vi "Test DI and DO.vi"() -> ()   [LabVIEW 2013]
uses:
  SLL DAQ Engine/Software/Source Code/Sub VIs/DAQ Engine/Controls/SLL DE List of Digital Inputs.ctl
  SLL DAQ Engine/Software/Source Code/Sub VIs/DAQ Engine/Controls/SLL DE List of Digital Outputs.ctl
  Controls/ALTS-2015 LV2GBL Station Info Options.ctl
  SLL DAQ Engine/Software/Source Code/Sub VIs/DAQ Engine/Controls/SLL DE DI Global Options.ctl
  SLL DAQ Engine/Software/Source Code/Sub VIs/DAQ Engine/Controls/SLL DE DO Global Options.ctl
panel:
  out "Station Number":string
  in  "PC_ACK_Read_Tags":dbl
  out "Test Type":i32
  out "DO Channel Name":T1
  out "String":string
  in  "Invalid_SNo":dbl
  in  "Station_No_Start_Stop_Test":dbl
  in  "Start_Test":dbl
  in  "Rerun":dbl
  in  "Station_Number":dbl
  in  "Test_Result":dbl
  in  "Serial_Flange_Size":string
  in  "Serial_Displacement_Size":dbl
  in  "Serial_Adapter_Size":dbl
  in  "New_Serial":dbl
  in  "Scan_Trigger":dbl
  in  "Stop_Test":dbl
  in  "Task_Available_for_Robot":dbl
  in  "Robot_Available":dbl
  in  "DI Array":bool[](array[boolean])=[FALSE, FALSE, FALSE, FALSE, FALSE, FALSE, FALSE, FALSE, FALSE, FALSE, FALSE, FALSE, FALSE, FALSE, FALSE, FALSE, FALSE, FALSE, FALSE, FALSE, FALSE, FALSE, FALSE, FALSE, FALSE, FALSE, FALSE, FALSE]
  in  "DI Channel Name Array":T2[](array[typedef])=[enum."STATION1_START", enum."STATION1_STOP", enum."STATION1_CLAMPED", enum."STATION1_TC_PASS", enum."STATION1_TC_FAIL", enum."STATION1_TTA", enum."STATION1_TTB", enum."STATION2_START", enum."STATION2_STOP", enum."STATION2_CLAMPED", enum."STATION2_TC_PASS", enum."STATION2_TC_FAIL", enum."STATION2_TTA", enum."STATION2_TTB", enum."STATION3_START", enum."STATION3_STOP", enum."STATION3_CLAMPED", enum."STATION3_TC_PASS", enum."STATION3_TC_FAIL", enum."STATION3_TTA", enum."STATION3_TTB", enum."STATION4_START", enum."STATION4_STOP", enum."STATION4_CLAMPED", enum."STATION4_TC_PASS", enum."STATION4_TC_FAIL", enum."STATION4_TTA", enum."STATION4_TTB"]
  out "DO Channel Name Array":T1[](array[typedef])=[enum."STATION1_START TEST", enum."STATION1_STOP TEST", enum."STATION1_LIGHT1", enum."STATION1_LIGHT2", enum."STATION1_LIGHT3", enum."STATION1_SELECT_TEST", enum."STATION2_START TEST", enum."STATION2_STOP TEST", enum."STATION2_LIGHT1", enum."STATION2_LIGHT2", enum."STATION2_LIGHT3", enum."STATION2_SELECT_TEST", enum."STATION3_START TEST", enum."STATION3_STOP TEST", enum."STATION3_LIGHT1", enum."STATION3_LIGHT2", enum."STATION3_LIGHT3", enum."STATION3_SELECT_TEST", enum."STATION4_START TEST", enum."STATION4_STOP TEST", enum."STATION4_LIGHT1", enum."STATION4_LIGHT2", enum."STATION4_LIGHT3", enum."STATION4_SELECT_TEST"]
  out "DO Status":bool[](array[boolean])
  out "error out":errorcluster
  in  "error in":errorcluster
  in  "DI Channel Name":T2
  in  "stop":bool
  # "Simulation VI to send DI Status and reads the DO output"
  # "Write Tags\nPC Writes to PLC\nPLC can only read these tags"
  # "Read Tags\nPC Reads from PLC"
  # "Test Type1: TTA:1, TTB: 0;\nTest Type2: TTA:0, TTB: 1;\nTest Type3: TTA:1, TTB: 1;\nTest Type4: TTA:0, TTB: 0;"
  # "IDLE : \t\t100\nTest Running:\t 010\nPass\t\t110\nFail\t\t101"
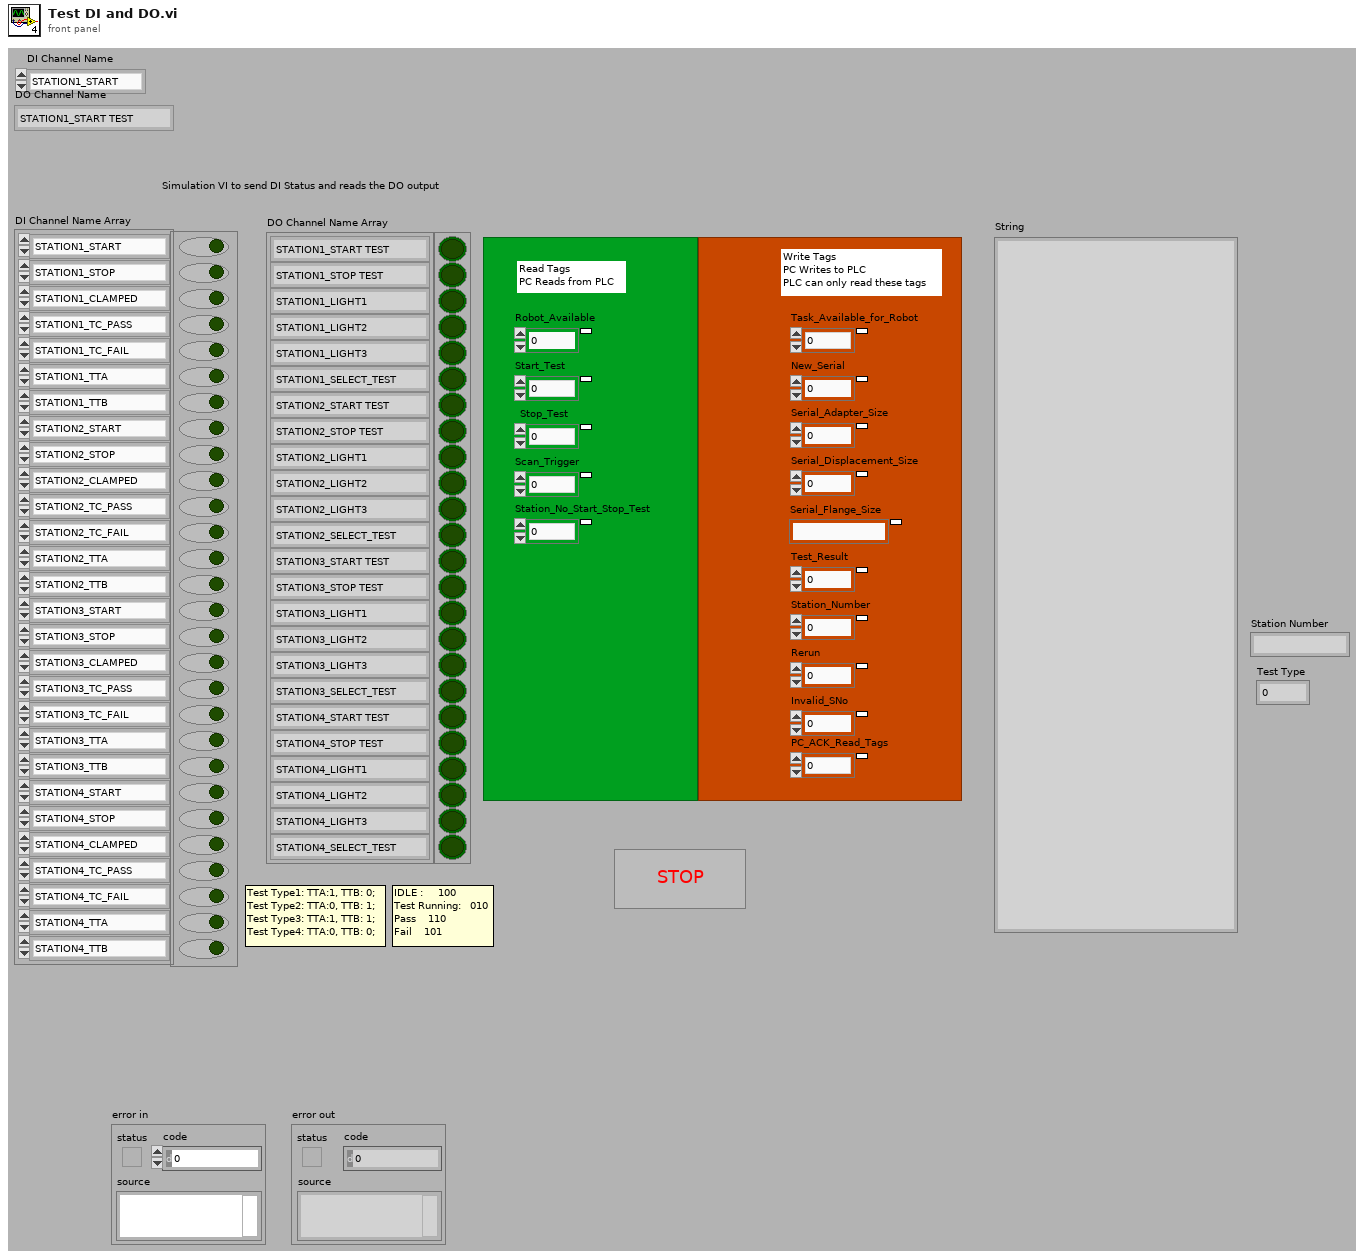
[diagram p1: front panel]
types:
  T1 = typedef "SLL DE List of Digital Outputs.ctl" = enum16{"STATION1_START TEST", "STATION1_STOP TEST", "STATION1_LIGHT1", "STATION1_LIGHT2", "STATION1_LIGHT3", "STATION1_SELECT_TEST", "STATION2_START TEST", "STATION2_STOP TEST", "STATION2_LIGHT1", "STATION2_LIGHT2", "STATION2_LIGHT3", "STATION2_SELECT_TEST", "STATION3_START TEST", "STATION3_STOP TEST", "STATION3_LIGHT1", "STATION3_LIGHT2", "STATION3_LIGHT3", "STATION3_SELECT_TEST", "STATION4_START TEST", "STATION4_STOP TEST", "STATION4_LIGHT1", "STATION4_LIGHT2", "STATION4_LIGHT3", "STATION4_SELECT_TEST"}
  T2 = typedef "SLL DE List of Digital Inputs.ctl" = enum16{"STATION1_START", "STATION1_STOP", "STATION1_CLAMPED", "STATION1_TC_PASS", "STATION1_TC_FAIL", "STATION1_TTA", "STATION1_TTB", "STATION2_START", "STATION2_STOP", "STATION2_CLAMPED", "STATION2_TC_PASS", "STATION2_TC_FAIL", "STATION2_TTA", "STATION2_TTB", "STATION3_START", "STATION3_STOP", "STATION3_CLAMPED", "STATION3_TC_PASS", "STATION3_TC_FAIL", "STATION3_TTA", "STATION3_TTB", "STATION4_START", "STATION4_STOP", "STATION4_CLAMPED", "STATION4_TC_PASS", "STATION4_TC_FAIL", "STATION4_TTA", "STATION4_TTB"}
  T3 = enum32{"No PSP", "Read", "Write", "Write & Read"}
  T4 = typedef "ALTS-2015 LV2GBL Station Info Options.ctl" = enum16{"Init", "Read", "Read All", "Write Sensor ID", "Write  Work Order", "Write Serial Number", "Write Test Data", "Write Station Status", "Write Station Occupancy", "Write Station Test Type", "Write Rerun", "Clear All", "Clear Test Result"}
  T5 = typedef "SLL DE DO Global Options.ctl" = enum16{"Init", "Write Line", "Write Array", "Write Full Status", "Read Line", "Read Array", "Read Full Status", "Restart DO", "Send to Safe Mode", "Stop DO"}
  T6 = typedef "SLL DE DI Global Options.ctl" = enum16{"Init", "Write Line", "Write Array", "Read Line", "Read Array", "Read Full Status", "Write Full Status"}
  T7 = typedef "ALTS-2015 Station Details.ctl" = cluster{"Station Number":string, "Work Order Number":string, "Sensor Name":string, "Pressure (PSI)":string, "Flow (SCCM)":string, "Test Time ":string, "Test Result":string, "Serial Number":string, "Station Status":T8, "Station Occupied?":bool, "Rerun Count":i32, "Test Type":i32}
  T8 = typedef "ALTS-2015 Status Ring Indicator.ctl" = u16
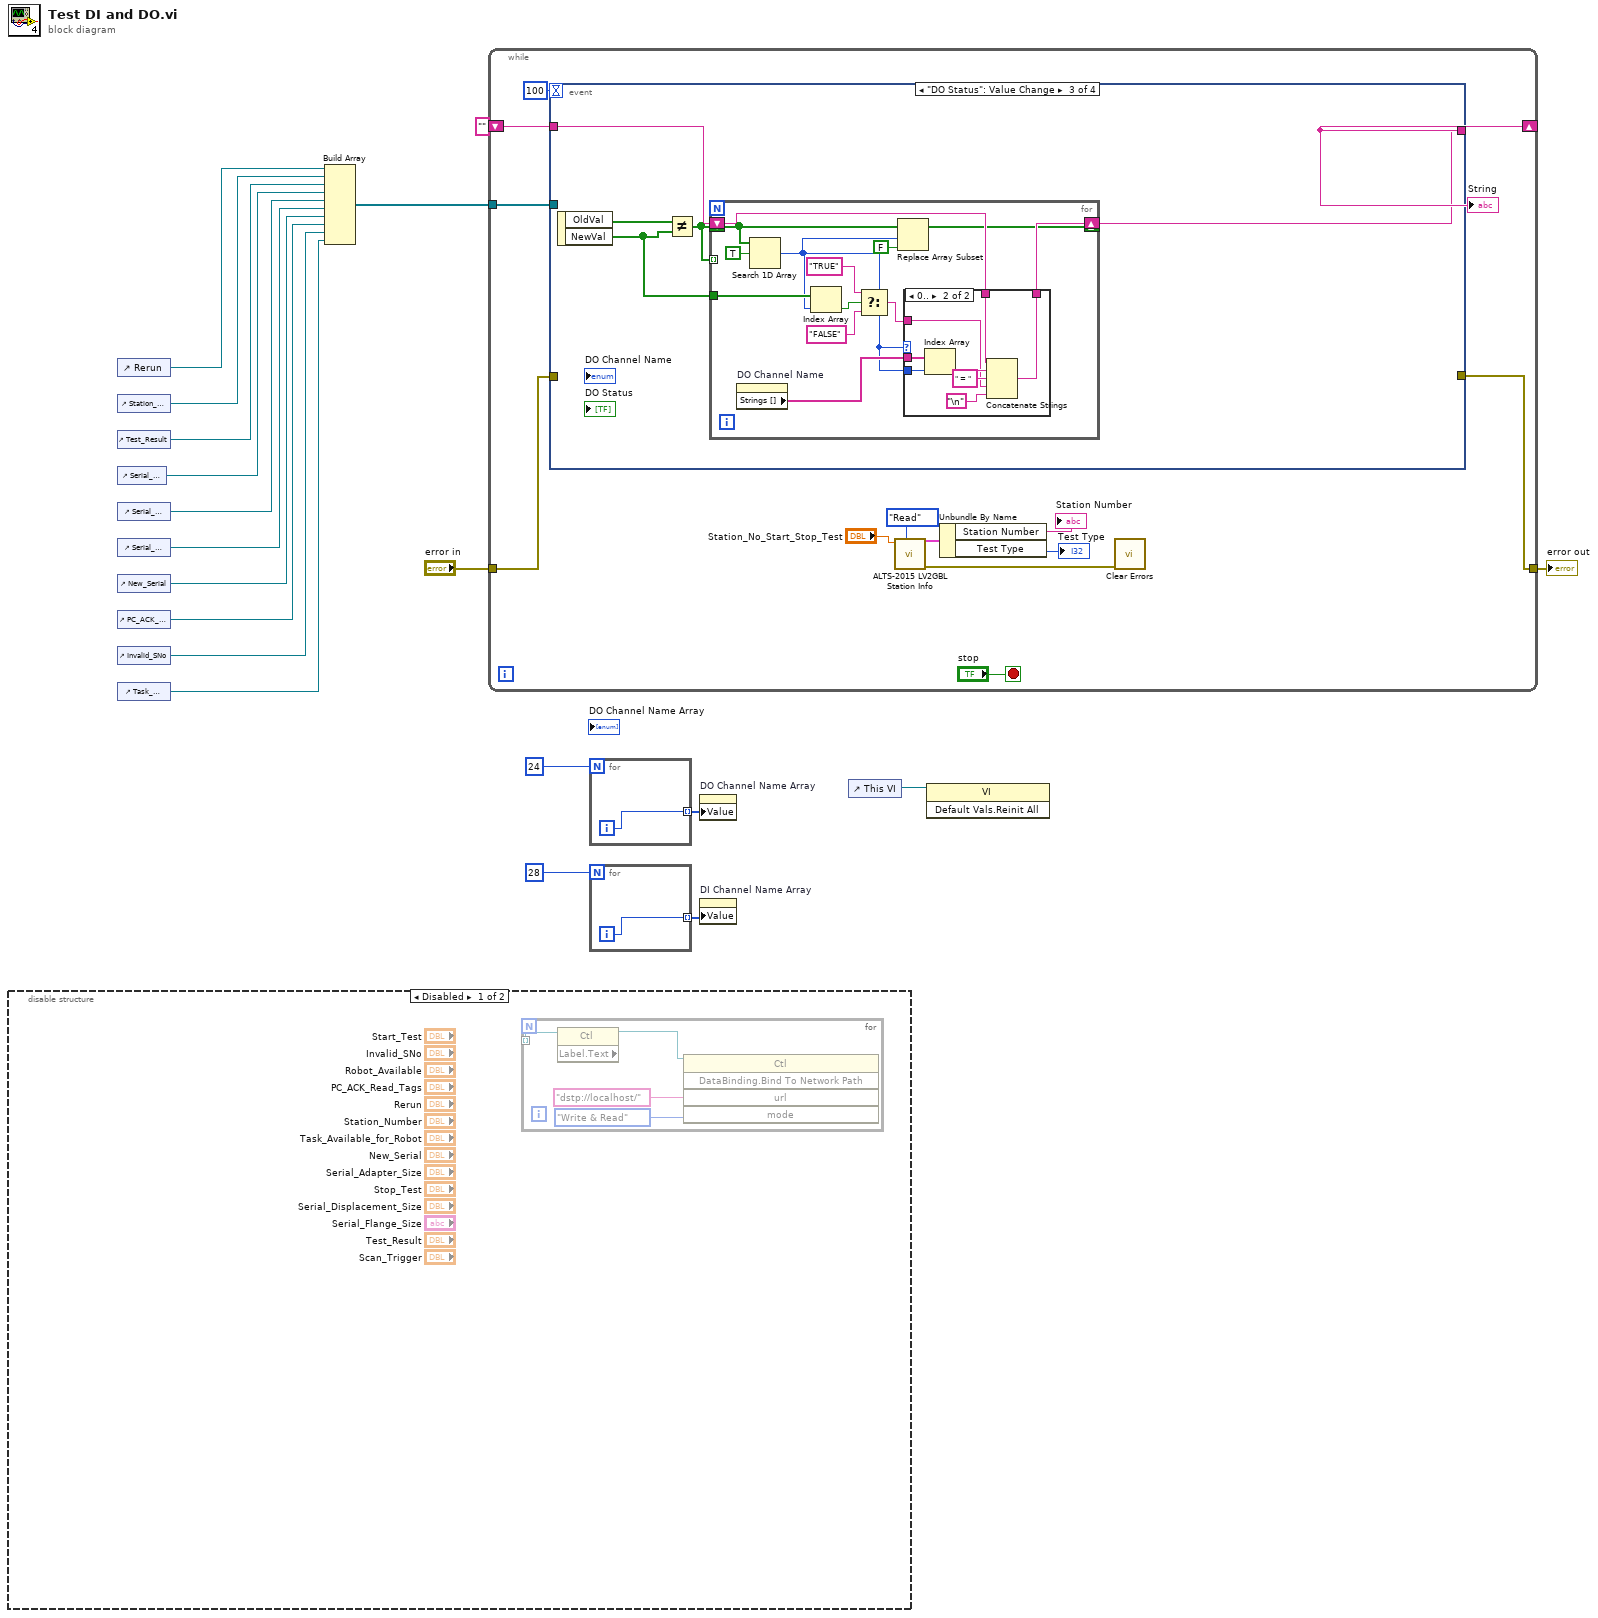
[diagram p0: block diagram]
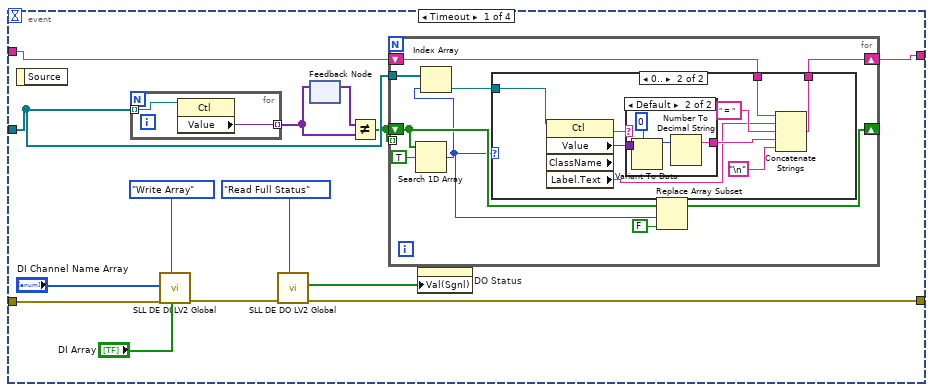
[diagram p3: hidden frame]
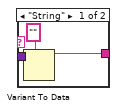
[diagram p5: hidden frame]
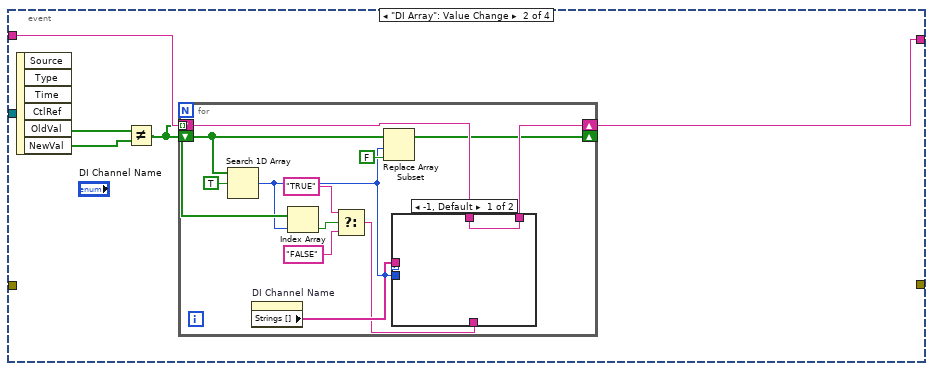
[diagram p6: hidden frame]
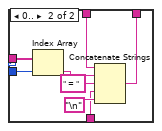
[diagram p7: hidden frame]
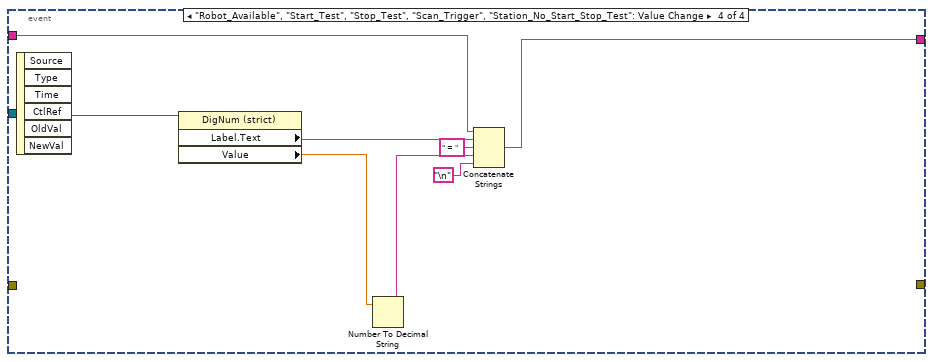
[diagram p9: hidden frame]
diagram:
  n1 = disable-structure shown="Disabled" {
    frame Disabled {
      n2 = for {
        tunnel: [w24] -> w20 mode=indexing
        n3 = property class="Ctl" props=["Label", "Text"](reference=w24) -> (reference out=w21:refnum<vi>)  [unwired: 1 in, 2 out]
        n4 = invoke on="Invoke Node" class="Ctl" method="DataBinding.Bind To Network Path"(reference=w21, "url"="dstp://localhost/" ("URL"), "mode"=T3."Write & Read" ("Mode")) -> ()  [unwired: 2 in, 5 out]
      }
    }
    frame Enabled {
    }
  }
  n5 = control-ref of="Rerun"() -> (w3:refnum<vi>)
  n6 = control-ref of="Station_Number"() -> (w4:refnum<vi>)
  n7 = control-ref of="Test_Result"() -> (w5:refnum<vi>)
  n8 = control-ref of="Serial_Flange_Size"() -> (w6:refnum<vi>)
  n9 = control-ref of="Serial_Displacement_Size"() -> (w7:refnum<vi>)
  n10 = control-ref of="Serial_Adapter_Size"() -> (w8:refnum<vi>)
  n11 = control-ref of="New_Serial"() -> (w9:refnum<vi>)
  n12 = control-ref of="PC_ACK_Read_Tags"() -> (w1:refnum<vi>)
  n13 = control-ref of="Invalid_SNo"() -> (w10:refnum<vi>)
  n14 = control-ref of="Task_Available_for_Robot"() -> (w11:refnum<vi>)
  n15 = Build Array(w3, w4, w5, w6, w7, w8, w9, w1, w10, w11) -> (w2:refnum<vi>[])
  n16 = while {
    tunnel: "error in" -> [w33]
    tunnel: [w32] -> w19
    shift-right: [w36] -> _
    shift-left: "" -> [w34]
    tunnel: w2 -> [w31]
    stop <- "stop" stop-if-true
    n17 = event shown="[2] \"DO Status\": Value Change" {
      selector: _ -> [_ _ _ _]
      dyn-events: _ -> [_ _ _ _]
      timeout: 100 -> [_ _ _ _]
      tunnel: [w39 w82 w109 w138] -> w36
      tunnel: w34 -> [w40 w81 w108 w139]
      tunnel: w33 -> [w45 _ _ _]
      tunnel: [w44 _ _ _] -> w32
      tunnel: w31 -> [w41 _ _ _]
      event Timeout {
        n18 = event-data() -> ()  [unwired: 1 in, 1 out]
        n19 = for {
          tunnel: w41 -> [w79] mode=indexing
          tunnel: [w78] -> w42 mode=indexing
          n20 = property class="Ctl"(reference=w79) -> ("Value"=w78:variant)  [unwired: 1 in, 2 out]
        }
        n21 = call "SLL DE DI LV2 Global.vi"("DI State Array"="DI Array", "Option"=SLL_DE_DI_Global_Options."Write Array", "error in (no error)"=w45, "DI Channel Name Array"="DI Channel Name Array") -> ("error out"=w50:errorcluster)  [unwired: 4 in, 3 out]
        n22 = call "SLL DE DO LV2 Global.vi"("DO Option"=SLL_DE_DO_Global_Options."Read Full Status", "Error In"=w50) -> ("error out"=w44:errorcluster, "Digital Array Status"=w51:bool[])  [unwired: 6 in, 2 out]
        n23 = feedback-in #1(w42) -> ()
        n24 = feedback #1() -> (w43:variant[])  [unwired: 1 in]
        n25 = Not Equal?(x=w43, y=w42) -> (x != y?=w38:bool[])
        n26 = for {
          tunnel: w41 -> [w59]
          shift-right: [w54] -> _
          shift-left: w38 -> [w55]
          tunnel: w38 -> [_] mode=indexing
          shift-right: [w57] -> w39
          shift-left: w40 -> [w58]
          n27 = Search 1D Array(1D array=w55, element=TRUE) -> (index of element=w53:i32)  [unwired: 1 in]
          n28 = Index Array(array=w59, index=w53) -> (element=w56:refnum<vi>)
          n29 = case shown="0.." w53 {
            tunnel: [w61 w69] -> w57
            tunnel: w58 -> [w61 w68]
            tunnel: w56 -> [_ w65]
            frame -1, Default {
            }
            frame 0.. {
              n30 = property class="Ctl"(reference=w65) -> ("Value"=w67:variant, "ClassName"=w64:string, "Label.Text"=w62:string)  [unwired: 1 in, 2 out]
              n31 = case shown="Default" w64 {
                tunnel: w67 -> [w72 w76]
                tunnel: [w71 w74] -> w66
                frame "String" {
                  n32 = Variant To Data(type="" ("concatenated string"), Variant=w72) -> (data=w71:string)  [unwired: 1 in, 1 out]
                }
                frame Default {
                  n33 = Variant To Data(type=0 ("concatenated string"), Variant=w76) -> (data=w75:i32)  [unwired: 1 in, 1 out]
                  n34 = Number To Decimal String(number=w75) -> (decimal integer string=w74:string)  [unwired: 1 in]
                }
              }
              n35 = Concatenate Strings(w68, w62, " = " ("string"), w66, "\n") -> (w69:string)
            }
          }
          n36 = Replace Array Subset(array=w55, new element=FALSE ("new element/subarray"), index=w53) -> (w54:bool[])
        }
        n37 = property on="DO Status" class="Arr (strict)"("Val(Sgnl)"=w51) -> ()  [unwired: 2 in, 2 out]
      }
      event "DI Array": Value Change {
        n38 = event-data() -> ("OldVal"=w84:bool[], "NewVal"=w83:bool[])  [unwired: 1 in, 4 out]
        n39 = Not Equal?(x=w84, y=w83) -> (x != y?=w80:bool[])
        n40 = for {
          tunnel: w80 -> [_] mode=indexing
          shift-right: [w88] -> _
          shift-left: w80 -> [w89]
          shift-right: [w94] -> w82
          shift-left: w81 -> [w93]
          n41 = Search 1D Array(1D array=w89, element=TRUE) -> (index of element=w85:i32)  [unwired: 1 in]
          n42 = property on="DI Channel Name" class="Enum (strict)"() -> ("Strings []"=w95:string[])  [unwired: 2 in, 2 out]
          n43 = Index Array(array=w89, index=w85) -> (element=w92:bool)
          n44 = Select(t="TRUE", s=w92, f="FALSE") -> (s? t:f=w86:string)
          n45 = Replace Array Subset(array=w89, new element=FALSE ("new element/subarray"), index=w85) -> (w88:bool[])
          n46 = case shown="-1, Default" w85 {
            tunnel: w95 -> [_ w105]
            tunnel: [w97 w103] -> w94
            tunnel: w93 -> [w97 w102]
            tunnel: w85 -> [_ w101]
            tunnel: w86 -> [_ w98]
            frame -1, Default {
            }
            frame 0.. {
              n47 = Index Array(array=w105, index=w101) -> (element=w104:string)
              n48 = Concatenate Strings(w102, w104, " = " ("string"), w98, "\n") -> (w103:string)
            }
          }
        }
      }
      event "DO Status": Value Change {
        n49 = event-data() -> ("OldVal"=w110:bool[], "NewVal"=w107:bool[])  [unwired: 1 in]
        n50 = Not Equal?(x=w110, y=w107) -> (x != y?=w106:bool[])
        n51 = for {
          tunnel: w107 -> [w119]
          tunnel: w106 -> [_] mode=indexing
          shift-right: [w113] -> _
          shift-left: w106 -> [w114]
          shift-right: [w122] -> w109
          shift-left: w108 -> [w121]
          n52 = property on="DO Channel Name" class="Enum (strict)"() -> ("Strings []"=w120:string[])  [unwired: 2 in, 2 out]
          n53 = Search 1D Array(1D array=w114, element=TRUE) -> (index of element=w112:i32)  [unwired: 1 in]
          n54 = Index Array(array=w119, index=w112) -> (element=w118:bool)
          n55 = Select(t="TRUE", s=w118, f="FALSE") -> (s? t:f=w115:string)
          n56 = Replace Array Subset(array=w114, new element=FALSE ("new element/subarray"), index=w112) -> (w113:bool[])
          n57 = case shown="0.." w112 {
            tunnel: w112 -> [_ w132]
            tunnel: [w124 w129] -> w122
            tunnel: w120 -> [_ w128]
            tunnel: w121 -> [w124 w127]
            tunnel: w115 -> [_ w125]
            frame -1, Default {
            }
            frame 0.. {
              n58 = Index Array(array=w128, index=w132) -> (element=w130:string)
              n59 = Concatenate Strings(w127, w130, " = " ("string"), w125, "\n") -> (w129:string)
            }
          }
        }
      }
      event "Robot_Available", "Start_Test", "Stop_Test", "Scan_Trigger", "Station_No_Start_Stop_Test": Value Change {
        n60 = event-data() -> ("CtlRef"=w140:refnum<vi>)  [unwired: 1 in, 5 out]
        n61 = property class="DigNum (strict)"(reference=w140) -> ("Label.Text"=w137:string, "Value"=w136:dbl)  [unwired: 1 in, 2 out]
        n62 = Number To Decimal String(number=w136) -> (decimal integer string=w135:string)  [unwired: 1 in]
        n63 = Concatenate Strings(w139, w137, " = " ("string"), w135, "\n") -> (w138:string)
      }
    }
    "String" <- w36
    n64 = call "ALTS-2015 LV2GBL Station Info.vi"("Options"=ALTS-2015_LV2GBL_Station_Info_Options."Read", "Station Cluster"="Station_No_Start_Stop_Test") -> ("error out"=w27:errorcluster, "Station Details"=w30:T7)  [unwired: 7 in, 1 out]
    n65 = Unbundle By Name(w30) -> ("Station Number"=→"Station Number":string, "Test Type"=→"Test Type":i32)
    n66 = call <vilib>:"Clear Errors.vi"("error in (no error)"=w27) -> ()  [unwired: 6 in, 1 out]
  }
  "error out" <- w19
  n67 = for {
    N: 24 -> [_]
    tunnel: [w141] -> w17 mode=indexing
    i -> [w141]
  }
  n68 = for {
    N: 28 -> [_]
    tunnel: [w142] -> w14 mode=indexing
    i -> [w142]
  }
  n69 = property on="DO Channel Name Array" class="Arr (strict)"("Value"=w17) -> ()  [unwired: 2 in, 2 out]
  n70 = property on="DI Channel Name Array" class="Arr (strict)"("Value"=w14) -> ()  [unwired: 2 in, 2 out]
  n71 = control-ref of="This VI"() -> (w13:refnum<vi>)
  n72 = invoke class="VI" method="Default Vals.Reinit All"(reference=w13) -> ()  [unwired: 2 in, 3 out]
